vi "ConfigureAnalogChannel.vi"(8 "error in (no error)":errorcluster, 11 "Oscilloscope in":refnum<class "Oscilloscope.lvclass">) -> (0 "error out":errorcluster, 3 "Oscilloscope out":refnum<class "Oscilloscope.lvclass">)   [LabVIEW 2020, in "Oscilloscope.lvclass"]
uses:
  Oscilloscope.lvclass
  C:/Code Projects/CircuitExplorer/AnalogDiscoveryFunction/AnalogDiscoveryFunction.lvclass
  AnalogDiscoveryFunction/AnalogDiscoveryFunction.lvclass/AnalogDiscoveryFunction.ctl
  AnalogDiscoveryFunction/GetInstrumentHandle.vi
  Oscilloscope.lvclass/Oscilloscope.ctl
  <vilib>/DigilentWF/DigilentWF.lvlib
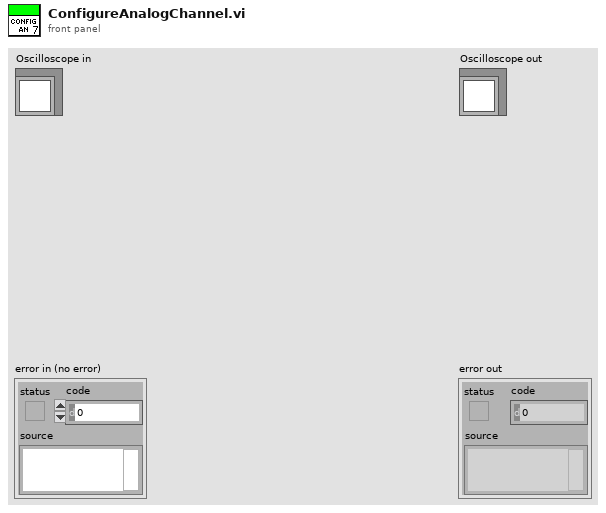
[diagram p1: front panel]
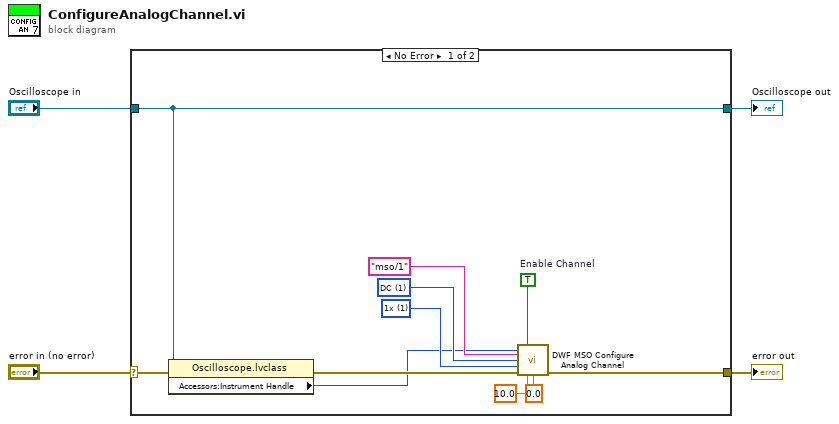
[diagram p0: block diagram]
diagram:
  n1 = case shown="No Error" "error in (no error)" {
    selector: "error in (no error)" -> [w10 w17]
    tunnel: [w15 w17] -> w3
    tunnel: [w8 w16] -> w1
    tunnel: "Oscilloscope in" -> [w8 w16]
    frame No Error {
      w11 = 1 items=["1x"=1, "10x"=10] ("Probe Attenuation")
      w12 = 1 items=["AC", "DC"] ("Vertical Coupling")
      w13 = TRUE  # Enable Channel
      n2 = property class="Oscilloscope.lvclass"(reference=w8, error in=w10) -> (error out=w9:errorcluster, "Accessors:Instrument Handle"=w7:u32)  [unwired: 1 out]
      n3 = call <vilib>:"DWF MSO Configure Analog Channel.vi"("Instrument Handle In"=w7, "Enable Channel"=w13, "Channel"="mso/1", "Vertical Coupling"=w12, "Probe Attenuation"=w11, "Error In"=w9, "Vertical Range"=10.0, "Vertical Offset"=0.0) -> ("Error Out"=w15:errorcluster)  [unwired: 6 in, 1 out]
    }
    frame Error {
    }
  }
  "error out" <- w3
  "Oscilloscope out" <- w1
